vi "Create_New_Build.vi"(6 "buildSpecName":string, 7 "Programmatic? (false)":bool, 8 "error in (no error)":errorcluster, 9 "buildObject":T1, 10 "Destination Path":path, 11 "AB_InteropAssembly in":refnum<class "AB_InteropAssembly.lvclass">) -> (0 "error out":errorcluster, 3 "AB_InteropAssembly out":refnum<class "AB_InteropAssembly.lvclass">)   [LabVIEW 2020, in "AB_InteropAssembly.lvclass"]
uses:
  <vilib>/AppBuilder/AB_Classes/InteropAssembly/AB_InteropAssembly.lvclass
  <resource>/Framework/Providers/API/ItemRef.ctl
  <vilib>/AppBuilder/AB_TargetFileType.ctl
  <vilib>/AppBuilder/AB_Classes/InteropAssembly/AB_InteropAssembly.lvclass/AB_InteropAssembly.ctl
  <resource>/Framework/Providers/Common/provcom_StringGlobals.vi
  <vilib>/AppBuilder/AB_Classes/Application/AB_Application.lvclass
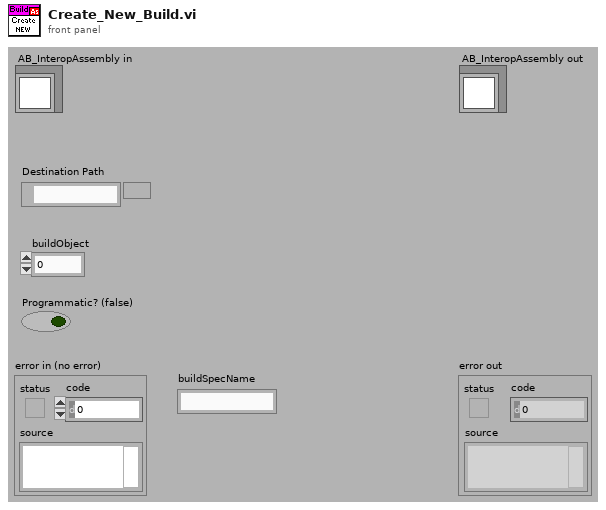
[diagram p1: front panel]
types:
  T1 = typedef "ItemRef.ctl" = u64
  T2 = typedef "AB_TargetFileType.ctl" = enum16{"EXE", "DLL", "RTEXE"}
  T3 = enum32{"invalid OS target", "Mac OS", "Windows 3.1", "Windows 95/NT", "Solaris 1", "Solaris 2", "HP-UX", "PowerMAX", "Linux", "Irix", "Rhapsody", "BeOS", "AIX", "OSF1", "VxWorks", "PharLap", "Carbon", "RTX", "Windows x64", "Linux x64", "Mac OS X x64"}
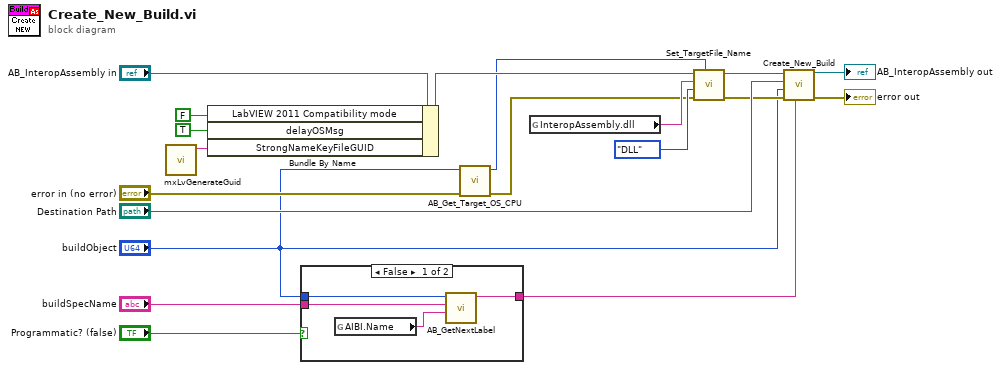
[diagram p0: block diagram]
diagram:
  n1 = call <resource>:"mxLvGenerateGuid.vi"() -> ("Value"=w15:string)  [unwired: 1 in, 10 out]
  n2 = Bundle By Name(cluster="AB_InteropAssembly in", "LabVIEW 2011 Compatibility mode"=FALSE ("data.LabVIEW 2011 Compatibility mode"), "delayOSMsg"=TRUE ("data.delayOSMsg"), "StrongNameKeyFileGUID"=w15) -> (w10:refnum<class "AB_InteropAssembly.lvclass">)
  n3 = case shown="False" "Programmatic? (false)" {
    tunnel: [w23 w24] -> w13
    tunnel: "buildSpecName" -> [w20 w24]
    tunnel: "buildObject" -> [w22 _]
    frame False {
      n4 = global read "provcom_StringGlobals.vi" "AIBI.Name"() -> (w21:string)
      n5 = call <vilib>:"AB_GetNextLabel.vi"("default name"=w21, "supplied name"=w20, "buildObject"=w22) -> ("New label"=w23:string)  [unwired: 2 in, 6 out]
    }
    frame True {
    }
  }
  n6 = call <resource>:"AB_Get_Target_OS_CPU.vi"("error in (no error)"="error in (no error)", "Object"="buildObject") -> ("error out"=w3:errorcluster, "Target Operating System"=w2:T3)  [unwired: 7 in, 1 out]
  n7 = global read "provcom_StringGlobals.vi" "InteropAssembly.dll"() -> (w7:string)
  n8 = call-dynamic "Set_TargetFile_Name.vi"("Target Operating System"=w2, "error in (no error)"=w3, "Target file type"=AB_TargetFileType."DLL" ("Build type"), "Target file name"=w7, "AB_Targetfile in"=w10) -> ("error out"=w8:errorcluster, "AB_Targetfile out"=w9:refnum<class "AB_InteropAssembly.lvclass">)  [unwired: 5 in]
  n9 = call-parent "Create_New_Build.vi"("buildSpecName"=w13, "error in (no error)"=w8, "buildObject"="buildObject", "Destination Path"="Destination Path", "AB_Application in"=w9) -> ("error out"=→"error out":errorcluster, "AB_Application out"=→"AB_InteropAssembly out":refnum<class "AB_InteropAssembly.lvclass">)  [unwired: 1 in, 4 out]
